vi "Pasco Drive Correcting.vi"(8 "RightDriveOutput":dbl, 11 "LeftDriveOutput":dbl) -> (0 "RightDriveOutput":dbl, 3 "LeftDriveOutput":dbl)   [LabVIEW 2011]
uses:
  Robot Global Data.vi
  <vilib>/addons/control/pid/pid.llb/PID (DBL).vi
  <vilib>/addons/control/pid/NI_PID_pid.lvlib
panel:
  in  "PID gains":T1={"proportional gain (Kc)"=1.0, "integral time (Ti, min)"=0.01, "derivative time (Td, min)"=0.0} {"derivative time (Td, min)" format="%.3f"; "integral time (Ti, min)" format="%.3f"; "proportional gain (Kc)" format="%.3f"}
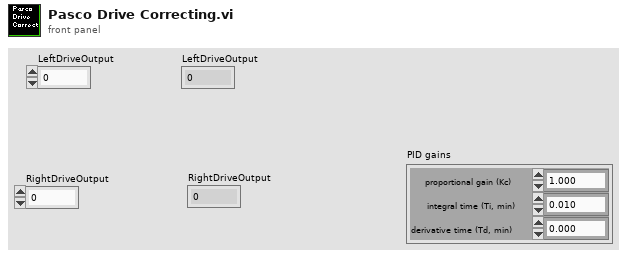
[diagram p1: front panel]
types:
  T1 = cluster{"proportional gain (Kc)":dbl, "integral time (Ti, min)":dbl, "derivative time (Td, min)":dbl}
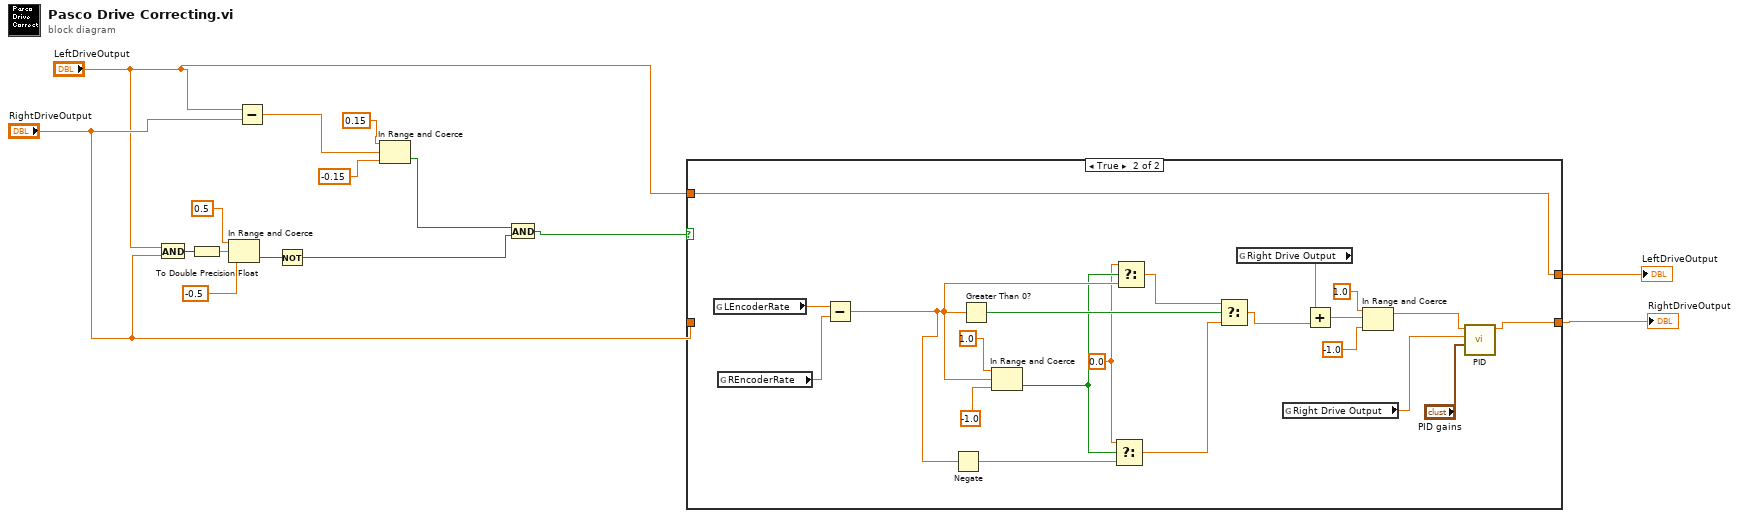
[diagram p0: block diagram]
diagram:
  n1 = And(x="LeftDriveOutput", y="RightDriveOutput") -> (x .and. y?=w10:i32)
  n2 = To Double Precision Float(number=w10) -> (double precision float=w9:dbl)
  n3 = In Range and Coerce(upper limit=0.5, x=w9, lower limit=-0.5) -> (In Range?=w6:bool)  [unwired: 1 out]
  n4 = Subtract(x="LeftDriveOutput", y="RightDriveOutput") -> (x-y=w13:dbl)
  n5 = Not(x=w6) -> (.not. x?=w5:bool)
  n6 = In Range and Coerce(upper limit=0.15, x=w13, lower limit=-0.15 ("upper limit")) -> (In Range?=w14:bool)  [unwired: 1 out]
  n7 = And(x=w14, y=w5) -> (x .and. y?=w15:bool)
  n8 = case shown="True" w15 {
    tunnel: [w17 w21] -> w3
    tunnel: "RightDriveOutput" -> [w17 _]
    tunnel: [w16 w18] -> w2
    tunnel: "LeftDriveOutput" -> [w16 w18]
    frame False {
    }
    frame True {
      w27 = 0.0
      n9 = global read "Robot Global Data.vi" "LEncoderRate"() -> (w38:dbl)
      n10 = global read "Robot Global Data.vi" "REncoderRate"() -> (w37:dbl)
      n11 = Subtract(x=w38, y=w37) -> (x-y=w30:dbl)
      n12 = Negate(x=w30) -> (-x=w31:dbl)
      n13 = Greater Than 0?(x=w30) -> (x > 0?=w36:bool)
      n14 = In Range and Coerce(upper limit=1.0, x=w30, lower limit=-1.0 ("upper limit")) -> (In Range?=w28:bool)  [unwired: 1 out]
      n15 = Select(t=w27, s=w28, f=w31) -> (s? t:f=w32:dbl)
      n16 = Select(t=w27, s=w28, f=w30) -> (s? t:f=w33:dbl)
      n17 = Select(t=w33, s=w36, f=w32) -> (s? t:f=w29:dbl)
      n18 = global read "Robot Global Data.vi" "Right Drive Output"() -> (w20:dbl)
      n19 = global read "Robot Global Data.vi" "Right Drive Output"() -> (w22:dbl)
      n20 = Add(x=w20, y=w29) -> (x+y=w26:dbl)
      n21 = In Range and Coerce(upper limit=1.0, x=w26, lower limit=-1.0 ("upper limit")) -> (coerced(x)=w23:dbl)  [unwired: 1 out]
      n22 = call-poly <vilib>:"PID.vi"("PID gains"="PID gains", "process variable"=w22, "setpoint"=w23) -> ("output"=w21:dbl)  [unwired: 7 in, 1 out]
    }
  }
  "LeftDriveOutput" <- w2
  "RightDriveOutput" <- w3
